vi "ConfigTrigger.vi"(8 "error in (no error)":errorcluster, 11 "NiPxi6123 in":refnum<class "NiPxi6123.lvclass">) -> (0 "error out":errorcluster, 3 "NiPxi6123 out":refnum<class "NiPxi6123.lvclass">)   [LabVIEW 2014, in "SamplerPlugins.lvlib" / "NiPxi6123.lvclass"]
uses:
  NiPxi6123.lvclass
  <vilib>/DAQmx/configure/trigger.llb/DAQmx Start Trigger (None).vi
  <vilib>/ErrorRing/Error Ring.xnode
  <vilib>/Utility/error.llb/Error Cluster From Error Code.vi
  <resource>/objmgr/daqmx.rc
  <vilib>/DAQmx/configure/trigger.llb/DAQmx Start Trigger (Digital Edge).vi
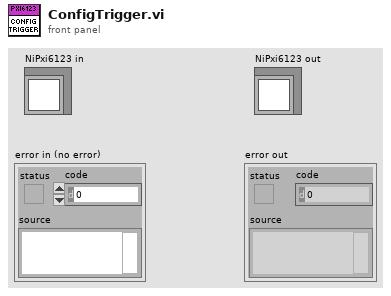
[diagram p1: front panel]
types:
  T1 = typedef "NISTSamplerPlugins.lvlib/NISTSamplerPluginsBase.lvclass/TriggerParams.ctl" = cluster{"eEdge":u16, "sSource":string}
  T2 = typedef "SamplerPlugins.lvlib/SamplerPluginsBase.lvclass/ConfigMultiPointParams.ctl" = cluster{"iTriggerCount":i32, "iSampleCount":i32, "eSampleClock":u16, "dSampleInterval":dbl}
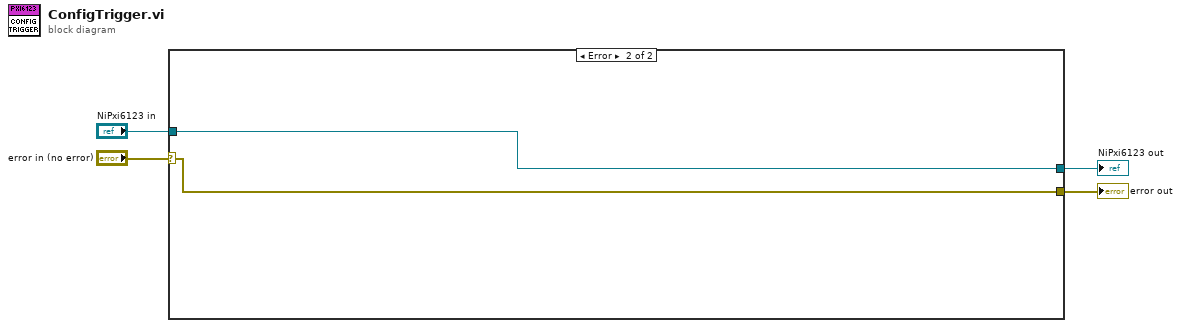
[diagram p0: block diagram]
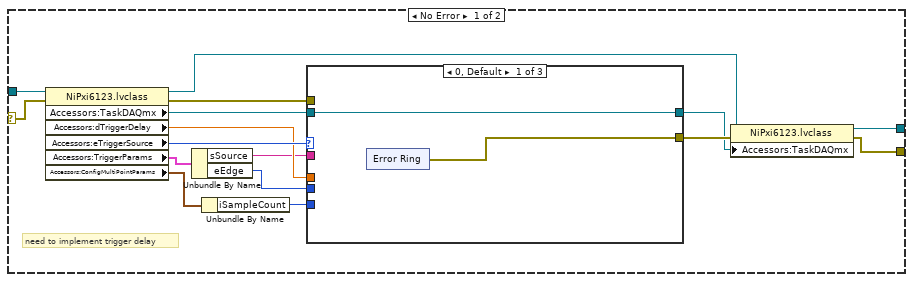
[diagram p2: hidden frame]
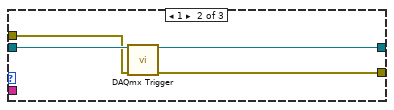
[diagram p3: hidden frame]
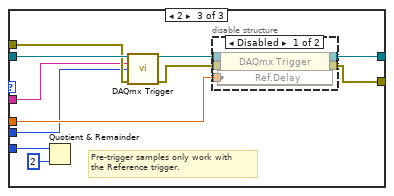
[diagram p4: hidden frame]
diagram:
  n1 = case shown="Error" "error in (no error)" {
    selector: "error in (no error)" -> [w19 w50]
    tunnel: "NiPxi6123 in" -> [w20 w51]
    tunnel: [w13 w51] -> w2
    tunnel: [w12 w50] -> w1
    frame No Error {
      # "need to implement trigger delay"
      n2 = property class="NiPxi6123.lvclass"(reference=w20, error in=w19) -> (reference out=w15:refnum<class "NiPxi6123.lvclass">, error out=w16:errorcluster, "Accessors:TaskDAQmx"=w17:refnum<k21>, "Accessors:dTriggerDelay"=w10:dbl, "Accessors:eTriggerSource"=w18:u16, "Accessors:TriggerParams"=w9:T1, "Accessors:ConfigMultiPointParams"=w6:T2)
      n3 = Unbundle By Name(w9) -> ("sSource"=w8:string, "eEdge"=w7:u16)
      n4 = Unbundle By Name(w6) -> ("iSampleCount"=w5:i32)
      n5 = case shown="0, Default" w18 {
        tunnel: [w22 w30 w36] -> w14
        tunnel: w17 -> [w21 w31 w42]
        tunnel: w16 -> [_ w29 w41]
        tunnel: [w21 w28 w37] -> w11
        tunnel: w10 -> [_ _ w38]
        tunnel: w8 -> [_ _ w35]
        tunnel: w7 -> [_ _ w34]
        tunnel: w5 -> [_ _ w33]
        frame 0, Default {
          n6 = xnode "Error Ring"() -> ("error out"=w22:errorcluster)
        }
        frame 1 {
          n7 = call-poly <vilib>:"DAQmx Trigger.vi"("task/channels in"=w31, "error in"=w29) -> ("task out"=w28:refnum<k21>, "error out"=w30:errorcluster)  [unwired: 12 in]
        }
        frame 2 {
          # "Pre-trigger samples only work with\nthe Reference trigger."
          n8 = Quotient & Remainder(x=w33, y=2) -> ()  [unwired: 2 out]
          n9 = call-poly <vilib>:"DAQmx Trigger.vi"("task/channels in"=w42, "source"=w35, "edge"=w34, "error in"=w41) -> ("task out"=w40:refnum<k21>, "error out"=w39:errorcluster)  [unwired: 10 in]
          n10 = disable-structure shown="Disabled" {
            disable-tunnel: w40 -> [w47 w49]
            disable-tunnel: w39 -> [w46 w48]
            disable-tunnel: w38 -> [w45 _]
            disable-tunnel: [w44 w49] -> w37
            disable-tunnel: [w43 w48] -> w36
            frame Disabled {
              n11 = property class="DAQmx Trigger"(reference=w47, error in=w46, "Ref.Delay"=w45) -> (reference out=w44:refnum<k21>, error out=w43:errorcluster)
            }
            frame Enabled {
            }
          }
        }
      }
      n12 = property class="NiPxi6123.lvclass"(reference=w15, error in=w14, "Accessors:TaskDAQmx"=w11) -> (reference out=w13:refnum<class "NiPxi6123.lvclass">, error out=w12:errorcluster)
    }
    frame Error {
    }
  }
  "error out" <- w1
  "NiPxi6123 out" <- w2
